vi "New Results.vi"(6 "Parameters":refnum<class "Analyze Parameter Base.lvclass">[](array[class]), 8 "error in (no error)":errorcluster, 9 "Image Nr.":i32, 10 "Results":refnum<class "Analyze Results Base.lvclass">[](array[class]), 11 "HIJ Vision Display in":refnum<class "HIJ Vision Display.lvclass">) -> (0 "error out":errorcluster, 3 "HIJ Vision Display out":refnum<class "HIJ Vision Display.lvclass">)   [LabVIEW 2020, in "HIJ Vision Display.lvlib" / "HIJ Vision Display.lvclass"]
uses:
  HIJ Vision Display.lvclass
  C:/Program Files (x86)/National Instruments/LabVIEW 2020/vi.lib/ActorFramework/Actor/Actor.lvclass
  Analyze/Results and Overlays/Results Base/Analyze Results Base.lvclass
  Analyze/Analyze Parameter/Analyze Parameter Base/Analyze Parameter Base.lvclass
  HIJ Vision Display.lvclass/HIJ Vision Display.ctl
  <vilib>/ActorFramework/Actor/Actor.lvclass/Actor.ctl
  Abstract Messages/Publish Analyze Results Msg/Publish Analyze Results Msg.lvclass/Publish Analyze Results Msg.ctl
  <vilib>/ActorFramework/Message Enqueuer/Message Enqueuer.lvclass/Message Enqueuer.ctl
  <vilib>/ActorFramework/Message Enqueuer/Enqueue.vi
  Abstract Messages/Publish Analyze Results Msg/Publish Analyze Results Msg.lvclass
  C:/Program Files (x86)/National Instruments/LabVIEW 2020/vi.lib/ActorFramework/Message/Message.lvclass
  <vilib>/ActorFramework/Message Priority Queue/Priority Enqueue.vi
  <vilib>/ActorFramework/Message Enqueuer/Message Enqueuer.lvclass
  Analyze/Results and Overlays/Static Overlay/Static Overlay.lvclass
  <vilib>/ActorFramework/Actor/Actor.lvclass
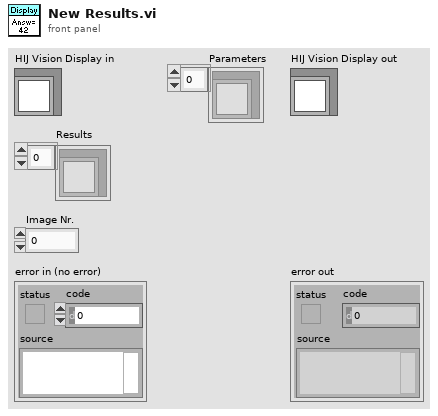
[diagram p1: front panel]
types:
  T1 = typedef "IMAQ Image.ctl" = refnum<image>
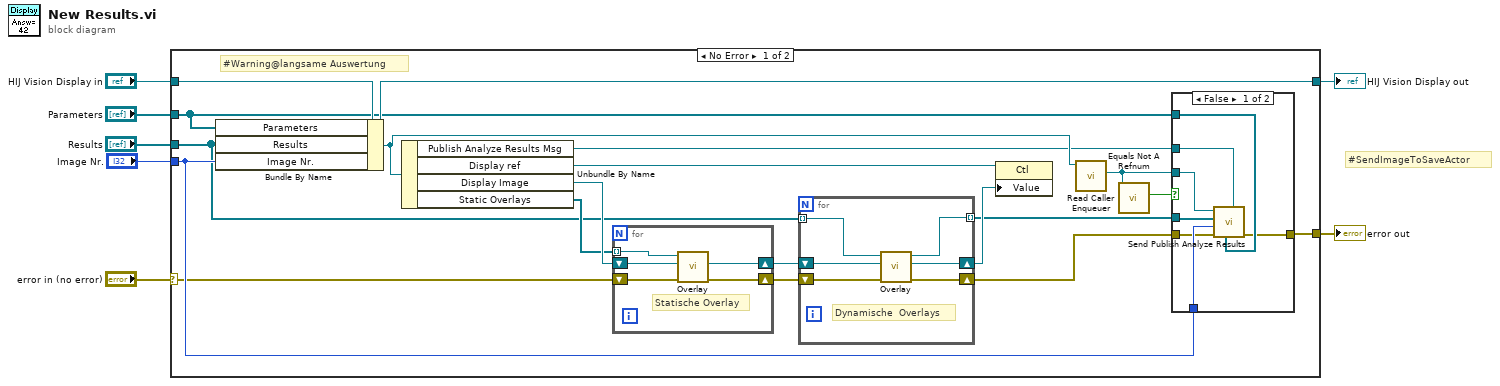
[diagram p0: block diagram]
diagram:
  # "#SendImageToSaveActor"
  n1 = case shown="No Error" "error in (no error)" {
    selector: "error in (no error)" -> [w10 w46]
    tunnel: [w14 w46] -> w6
    tunnel: [w23 w45] -> w4
    tunnel: "HIJ Vision Display in" -> [w25 w45]
    tunnel: "Results" -> [w8 _]
    tunnel: "Image Nr." -> [w13 _]
    tunnel: "Parameters" -> [w22 _]
    frame No Error {
      # "#Warning@langsame Auswertung"
      n2 = Bundle By Name(cluster=w25, "Parameters"=w22, "Results"=w8, "Image Nr."=w13) -> (w23:refnum<class "HIJ Vision Display.lvclass">)
      n3 = Unbundle By Name(w23) -> ("Publish Analyze Results Msg"=w16:refnum<class "Publish Analyze Results Msg.lvclass">, "Display ref"=w21:refnum<vi>, "Display Image"=w24:T1, "Static Overlays"=w12:refnum<class "Static Overlay.lvclass">[])
      n4 = for {
        tunnel: w12 -> [w30] mode=indexing
        shift-right: [w28] -> w11
        shift-left: w24 -> [w29]
        shift-right: [w26] -> w9
        shift-left: w10 -> [w27]
        # "Statische Overlay"
        n5 = call-dynamic "Overlay.vi"("error in (no error)"=w27, "Image In"=w29, "Overlay Base in"=w30) -> ("error out"=w26:errorcluster, "Image out"=w28:T1)  [unwired: 6 in, 1 out]
      }
      n6 = for {
        shift-right: [w43] -> w20
        shift-left: w11 -> [w40]
        tunnel: w8 -> [w44] mode=indexing
        tunnel: [w42] -> w17 mode=indexing
        shift-right: [w41] -> w15
        shift-left: w9 -> [w39]
        # "Dynamische  Overlays"
        n7 = call-dynamic "Overlay.vi"("error in (no error)"=w39, "Image In"=w40, "Overlay Base in"=w44) -> ("error out"=w41:errorcluster, "Image out"=w43:T1, "Overlay Base out"=w42:refnum<class "Analyze Results Base.lvclass">)  [unwired: 6 in]
      }
      n8 = property class="Ctl"(reference=w21, "Value"=w20) -> ()  [unwired: 1 in, 2 out]
      n9 = call <vilib>:"Read Caller Enqueuer.vi"("Actor"=w23) -> ("Caller Enqueuer"=w18:refnum<class "Message Enqueuer.lvclass">)  [unwired: 10 in]
      n10 = call <vilib>:"Equals Not A Refnum.vi"("Message Enqueuer"=w18) -> ("Not a refnum?"=w19:bool)  [unwired: 10 in]
      n11 = case shown="False" w19 {
        tunnel: w18 -> [w36 _]
        tunnel: w17 -> [w35 _]
        tunnel: w22 -> [w34 _]
        tunnel: w16 -> [w33 _]
        tunnel: w15 -> [w32 w38]
        tunnel: [w31 w38] -> w14
        tunnel: w13 -> [w37 _]
        frame False {
          n12 = call "Send Publish Analyze Results.vi"("Message Type"=w33, "Parameters"=w34, "error in (no error)"=w32, "Image Nr."=w37, "Results In"=w35, "Message Enqueuer"=w36) -> ("error out"=w31:errorcluster)  [unwired: 4 in, 1 out]
        }
        frame True {
        }
      }
    }
    frame Error {
    }
  }
  "error out" <- w6
  "HIJ Vision Display out" <- w4
